vi "Count AE.vi"(1 "Register":bool, 2 "Unregister":bool) -> (0 "Count":u32)   [LabVIEW 2025]
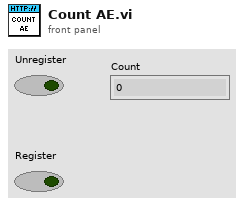
[diagram p1: front panel]
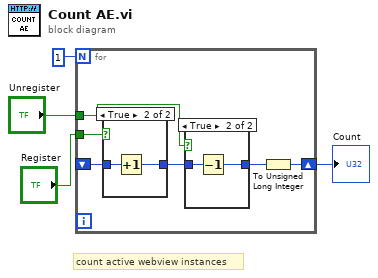
[diagram p0: block diagram]
diagram:
  # "count active webview instances"
  n1 = for {
    N: 1 -> [_]
    tunnel: "Register" -> [w7]
    tunnel: "Unregister" -> [w5]
    shift-right: [w8] -> w2
    shift-left: _ -> [w9]
    n2 = case shown="True" w7 {
      tunnel: [w14 w16] -> w10
      tunnel: w9 -> [w14 w15]
      frame False {
      }
      frame True {
        n3 = Increment(x=w15) -> (x+1=w16:u32)
      }
    }
    n4 = case shown="True" w5 {
      tunnel: w10 -> [w11 w13]
      tunnel: [w11 w12] -> w6
      frame False {
      }
      frame True {
        n5 = Decrement(x=w13) -> (x-1=w12:u32)
      }
    }
    n6 = To Unsigned Long Integer(number=w6) -> (unsigned 32bit integer=w8:u32)
  }
  "Count" <- w2
